vi "Configure Harmonics.vi"(5 "Current Harmonic Range (7)":dbl=7.0 caption="Current Harmonics Range (7)" min=1.0 max=50.0 step=1.0, 7 "Voltage Harmonic Range (7)":dbl=7.0 caption="Voltage Harmonics Range (7)" min=1.0 max=50.0 step=1.0, 8 "error in (no error)":errorcluster, 9 "Current Harmonic Sequence (Odd & Even)":u16(ring) items=["Odd & Even", "Odd Only"], 10 "Voltage Harmonic Sequence (Odd & Even)":u16(ring) items=["Odd & Even", "Odd Only"], 11 "VISA resource name":refnum<visa-resource-name>) -> (0 "error out":errorcluster, 3 "VISA resource name out":refnum<visa-resource-name>)   [LabVIEW 2015, in "Voltech PM1000+.lvlib"]
doc: "Configures both voltage and current scaling factors. It also indicates the voltage and current scaling factors.\n\nA current transformer produces an output current which is proportional to the load\ncurrent being measured. For example, the Voltech CL100 produces an output current\nthat is 1/100 of the current being measured.\nTo measure the correct current on the PM1000+, use the scale function of the analyzer\nto scale, or multiply, the CT output current.\nFor example, the CL100 is a 100:1 CT. When measuring 100A, its output is 1A. To\nscale this on the PM1000+, a scale factor of 100 must be entered. And PM1000+ is now ready to make measurements using a CT."
uses:
  <instrlib>/Voltech PM1000+/Voltech PM1000+.lvlib
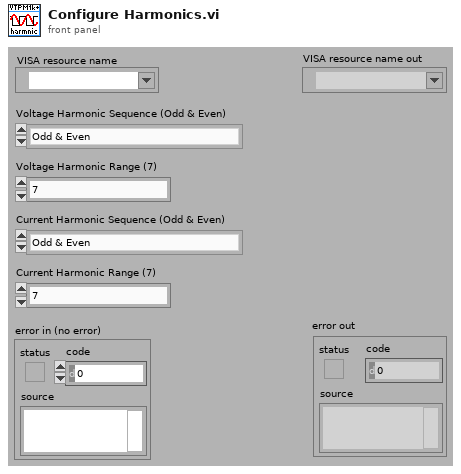
[diagram p1: front panel]
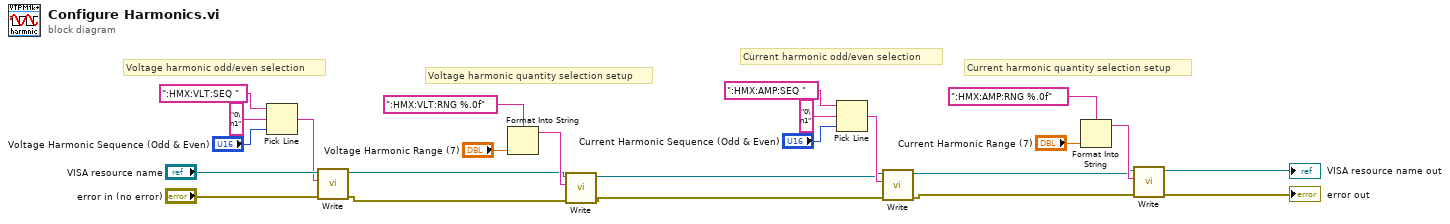
[diagram p0: block diagram]
diagram:
  # "Current harmonic quantity selection setup"
  # "Current harmonic odd/even selection"
  # "Voltage harmonic quantity selection setup"
  # "Voltage harmonic odd/even selection"
  n1 = Pick Line(string ("")=":HMX:VLT:SEQ ", multi-line string="0\n1", line index="Voltage Harmonic Sequence (Odd & Even)") -> (output string=w9:string)
  n2 = call <instrlib>:"Write.vi"("error in (no error)"="error in (no error)", "Write Buffer"=w9, "VISA resource name"="VISA resource name") -> ("error out"=w7:errorcluster, "VISA resource name out"=w8:refnum<visa-resource-name>)  [unwired: 7 in]
  n3 = Format Into String(format string=":HMX:VLT:RNG %.0f", "Voltage Harmonic Range (7)") -> (resulting string=w10:string)  [unwired: 2 in, 1 out]
  n4 = call <instrlib>:"Write.vi"("error in (no error)"=w7, "Write Buffer"=w10, "VISA resource name"=w8) -> ("error out"=w5:errorcluster, "VISA resource name out"=w6:refnum<visa-resource-name>)  [unwired: 7 in]
  n5 = Pick Line(string ("")=":HMX:AMP:SEQ ", multi-line string="0\n1", line index="Current Harmonic Sequence (Odd & Even)") -> (output string=w11:string)
  n6 = call <instrlib>:"Write.vi"("error in (no error)"=w5, "Write Buffer"=w11, "VISA resource name"=w6) -> ("error out"=w3:errorcluster, "VISA resource name out"=w4:refnum<visa-resource-name>)  [unwired: 7 in]
  n7 = Format Into String(format string=":HMX:AMP:RNG %.0f", "Current Harmonic Range (7)") -> (resulting string=w12:string)  [unwired: 2 in, 1 out]
  n8 = call <instrlib>:"Write.vi"("error in (no error)"=w3, "Write Buffer"=w12, "VISA resource name"=w4) -> ("error out"=→"error out":errorcluster, "VISA resource name out"=→"VISA resource name out":refnum<visa-resource-name>)  [unwired: 7 in]
